vi "createLEDParaArray.vi"(1 "ParaCluster":T1) -> (0 "ledParaArray":i32[](array[numeric]) format="%_2f")   [LabVIEW 2014]
uses:
  ParaCluster_def.ctl
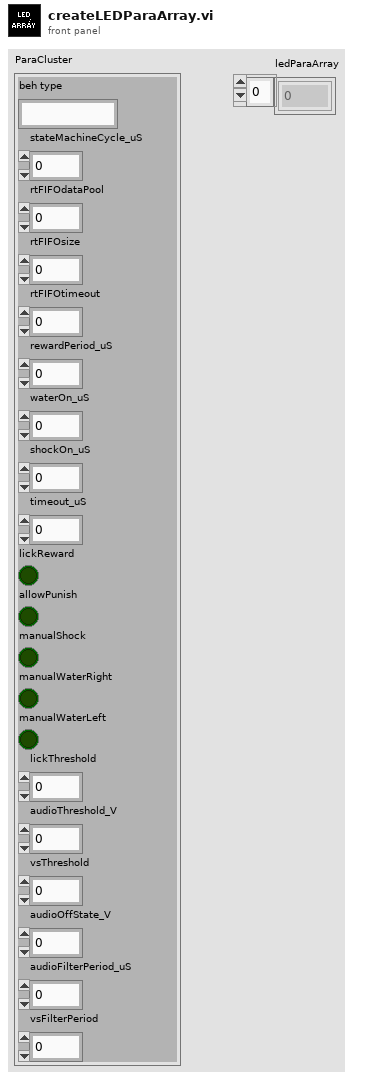
[diagram p1: front panel]
types:
  T1 = typedef "ParaCluster_def.ctl" = cluster{"beh type":string, "stateMachineCycle_uS":u32, "rtFIFOdataPool":u32, "rtFIFOsize":u32, "rtFIFOtimeout":u32, "rewardPeriod_uS":u32, "waterOn_uS":u32, "shockOn_uS":u32, "timeout_uS":u32, "lickReward":bool, "allowPunish":bool, "manualShock":bool, "manualWaterRight":bool, "manualWaterLeft":bool, "lickThreshold":fxp<+/-,16,5>, "audioThreshold_V":fxp<+/-,16,5>, "vsThreshold":fxp<+/-,16,5>, "audioOffState_V":fxp<+/-,16,5>, "audioFilterPeriod_uS":i32, "vsFilterPeriod":i32}
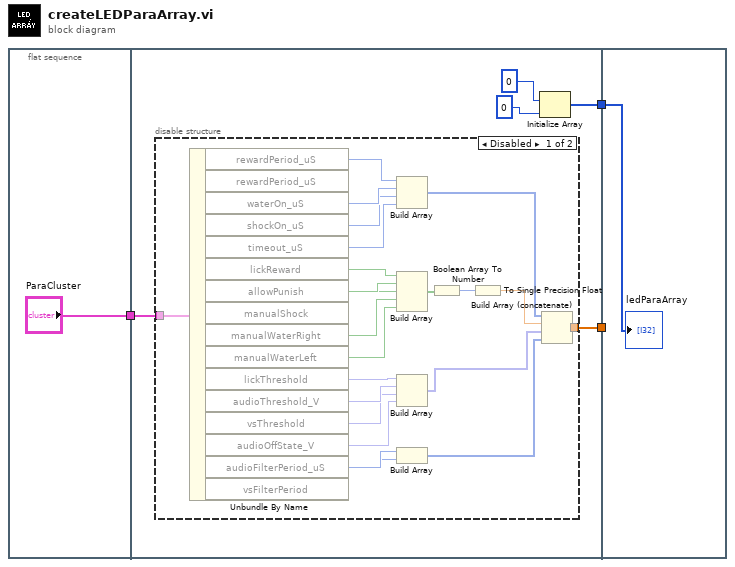
[diagram p0: block diagram]
diagram:
  n1 = flat-sequence {
    tunnel: ["ParaCluster"] -> w2
    tunnel: [w9] -> w3
    tunnel: w2 -> [w8]
    tunnel: [w6] -> w1
    tunnel: w3 -> [_]
    tunnel: w1 -> [w33]
    frame #0 {
    }
    frame #1 {
      n2 = disable-structure shown="Disabled" {
        disable-tunnel: [w11 _] -> w9
        disable-tunnel: w8 -> [w10 _]
        frame Disabled {
          n3 = Unbundle By Name(w10) -> ("rewardPeriod_uS"=w32:u32, "waterOn_uS"=w31:u32, "shockOn_uS"=w30:u32, "timeout_uS"=w29:u32, "lickReward"=w28:bool, "allowPunish"=w27:bool, "manualShock"=w26:bool, "manualWaterRight"=w25:bool, "manualWaterLeft"=w24:bool, "lickThreshold"=w23:fxp<+/-,16,5>, "audioThreshold_V"=w22:fxp<+/-,16,5>, "vsThreshold"=w21:fxp<+/-,16,5>, "audioOffState_V"=w20:fxp<+/-,16,5>, "audioFilterPeriod_uS"=w19:i32, "vsFilterPeriod"=w18:i32)  [unwired: 1 out]
          n4 = Build Array(w32, w31, w30, w29) -> (w15:u32[])
          n5 = Build Array ("para")(w28, w27, w26, w25, w24) -> (w17:bool[])
          n6 = Build Array ("para")(w23, w22, w21, w20) -> (w13:fxp<+/-,16,5>[])
          n7 = Build Array ("para")(w19, w18) -> (w12:i32[])
          n8 = Boolean Array To Number(Boolean array=w17) -> (number=w16:u32)
          n9 = To Single Precision Float(number=w16) -> (single precision float=w14:sgl)
          n10 = Build Array (concatenate)(w15, w14, w13, w12) -> (w11:sgl[])
        }
        frame Enabled {
        }
      }
      n11 = Initialize Array(0, 0) -> (w6:i32[])
    }
    frame #2 {
      "ledParaArray" <- w33
    }
  }
